vi "VerifStates.vi"(8 "error in (no error)":errorcluster, 11 "Instrument in":refnum<class "Instrument.lvclass">) -> (0 "error out":errorcluster, 3 "Instrument out":refnum<class "Instrument.lvclass">)   [LabVIEW 2018, in "Instrument.lvclass"]
uses:
  Instrument.lvclass
  Instrument.lvclass/Instrument.ctl
  Device/Optics/Opt_Selector/Opt_Selector.lvclass
  Device/Optics/Opt_Continuous/Opt_Continuous.lvclass
  StateMachine/State Machine.lvclass
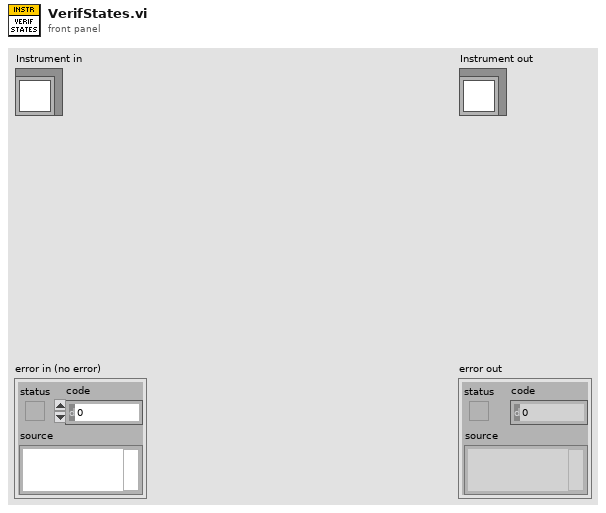
[diagram p1: front panel]
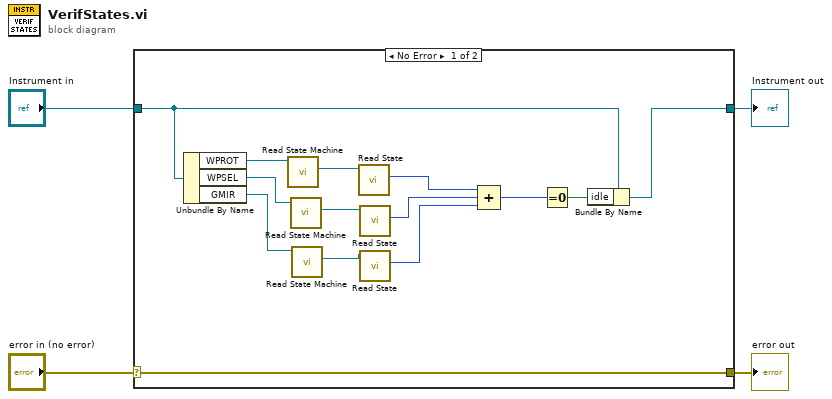
[diagram p0: block diagram]
diagram:
  n1 = case shown="No Error" "error in (no error)" {
    selector: "error in (no error)" -> [w18 w20]
    tunnel: [w18 w20] -> w3
    tunnel: [w9 w19] -> w1
    tunnel: "Instrument in" -> [w12 w19]
    frame No Error {
      n2 = Unbundle By Name(w12) -> ("WPROT"=w17:refnum<class "Opt_Selector.lvclass">, "WPSEL"=w6:refnum<class "Opt_Selector.lvclass">, "GMIR"=w5:refnum<class "Opt_Continuous.lvclass">)
      n3 = call-dynamic "Read State Machine.vi"("Device in"=w17) -> ("State Machine.lvclass"=w16:refnum<class "State Machine.lvclass">)  [unwired: 8 in, 2 out]
      n4 = call-dynamic "Read State Machine.vi"("Device in"=w6) -> ("State Machine.lvclass"=w8:refnum<class "State Machine.lvclass">)  [unwired: 8 in, 2 out]
      n5 = call-dynamic "Read State Machine.vi"("Device in"=w5) -> ("State Machine.lvclass"=w7:refnum<class "State Machine.lvclass">)  [unwired: 8 in, 2 out]
      n6 = call-dynamic "Read State.vi"("State Machine in"=w16) -> ("State"=w15:i32)  [unwired: 8 in, 2 out]
      n7 = call-dynamic "Read State.vi"("State Machine in"=w8) -> ("State"=w14:i32)  [unwired: 8 in, 2 out]
      n8 = call-dynamic "Read State.vi"("State Machine in"=w7) -> ("State"=w13:i32)  [unwired: 8 in, 2 out]
      n9 = Compound Arithmetic op=ADD(w15, w14, w13) -> (w10:i32)
      n10 = Equal To 0?(x=w10) -> (x = 0?=w11:bool)
      n11 = Bundle By Name(cluster=w12, "idle"=w11) -> (w9:refnum<class "Instrument.lvclass">)
    }
    frame Error {
    }
  }
  "error out" <- w3
  "Instrument out" <- w1
